vi "robotModeCtor.vi"(8 "error in (no error)":errorcluster, 10 "Allowed Robot Modes":string[](array[string]), 11 "Name":string) -> (0 "error out":errorcluster, 3 "Command out":refnum<class "Command.lvclass">)   [LabVIEW 2017, in "Command.lvclass"]
uses:
  <userlib>/836-Library/Robot/Command/Command.lvclass
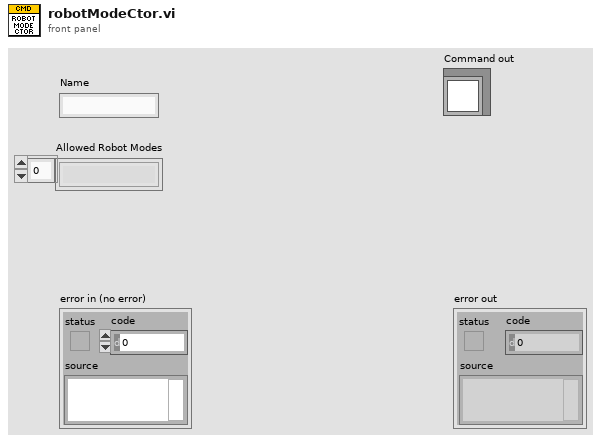
[diagram p1: front panel]
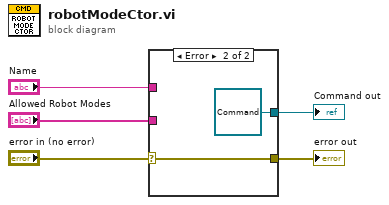
[diagram p0: block diagram]
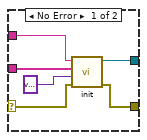
[diagram p2: hidden frame]
diagram:
  n1 = case shown="Error" "error in (no error)" {
    selector: "error in (no error)" -> [w8 w13]
    tunnel: [w7 w13] -> w4
    tunnel: "Name" -> [w11 _]
    tunnel: "Allowed Robot Modes" -> [w10 _]
    tunnel: [w6 refnum<class "Command.lvclass"> refnum ("Command out")] -> w1
    frame No Error {
      n2 = call <userlib>:"init.vi"("error in (no error)"=w8, "Default Data"=variant, "Allowed Robot Modes"=w10, "Name"=w11) -> ("error out"=w7:errorcluster, "Command out"=w6:refnum<class "Command.lvclass">)  [unwired: 6 in]
    }
    frame Error {
    }
  }
  "error out" <- w4
  "Command out" <- w1
